vi "Calculate the Apriltag Squares Center Location.vi"(10 "Pixels":i32=8) -> (2 "Array 2":i32[](array[numeric]))   [LabVIEW 2025]
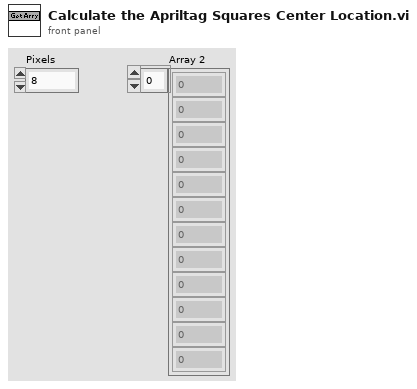
[diagram p1: front panel]
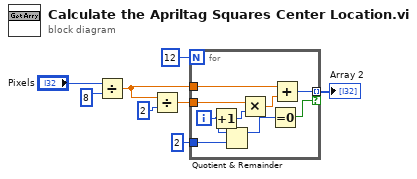
[diagram p0: block diagram]
diagram:
  n1 = Divide(x="Pixels", y=8) -> (x/y=w6:sgl)
  n2 = Divide(x=w6, y=2) -> (x/y=w5:sgl)
  n3 = for {
    N: 12 -> [_]
    tunnel: [w17] -> w4 mode=indexing if=w10
    tunnel: w5 -> [w16]
    tunnel: w6 -> [w13]
    tunnel: 2 ("y") -> [w9]
    i -> [w12]
    n4 = Increment(x=w12) -> (x+1=w14:i32)
    n5 = Quotient & Remainder(x=w12, y=w9) -> (x-y*floor(x/y)=w11:i32)  [unwired: 1 out]
    n6 = Multiply(x=w16, y=w14) -> (x*y=w15:sgl)
    n7 = Equal To 0?(x=w11) -> (x = 0?=w10:bool)
    n8 = Add(x=w13, y=w15) -> (x+y=w17:i32)
  }
  "Array 2" <- w4
